vi "Untitled 2.vi"() -> ()   [LabVIEW 2010]
panel:
  in  "VISA resource name":refnum<visa-resource-name>
  out "VISA resource name out":refnum<visa-resource-name>
  out "error out":errorcluster
  in  "error in (no error)":errorcluster
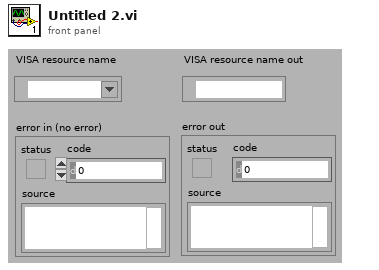
[diagram p1: front panel]
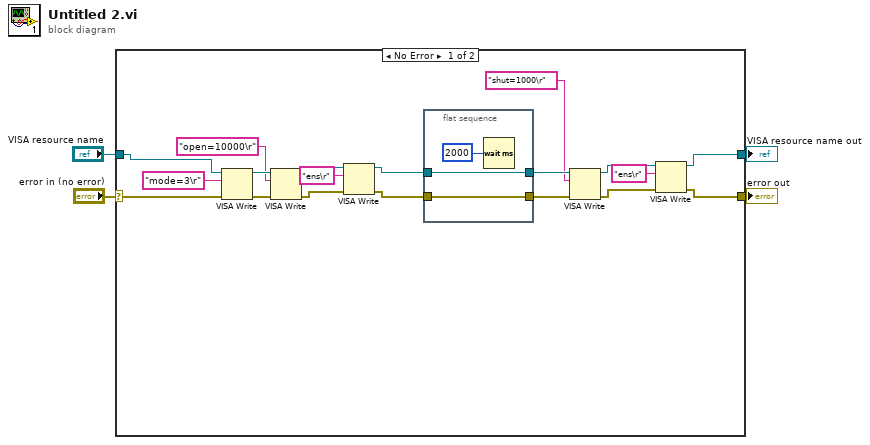
[diagram p0: block diagram]
diagram:
  n1 = case shown="No Error" "error in (no error)" {
    selector: "error in (no error)" -> [w23 w27]
    tunnel: [w6 w27] -> w3
    tunnel: [w8 w28] -> w2
    tunnel: "VISA resource name" -> [w22 w28]
    frame No Error {
      n2 = VISA Write(VISA resource name=w22, write buffer="mode=3\r", error in (no error)=w23) -> (VISA resource name out=w20:refnum<visa-resource-name>, error out=w19:errorcluster)  [unwired: 1 out]
      n3 = VISA Write(VISA resource name=w20, write buffer="open=10000\r", error in (no error)=w19) -> (VISA resource name out=w14:refnum<visa-resource-name>, error out=w13:errorcluster)  [unwired: 1 out]
      n4 = VISA Write(VISA resource name=w14, write buffer="ens\r", error in (no error)=w13) -> (VISA resource name out=w11:refnum<visa-resource-name>, error out=w12:errorcluster)  [unwired: 1 out]
      n5 = flat-sequence {
        tunnel: w11 -> [w25]
        tunnel: [w25] -> w17
        tunnel: w12 -> [w24]
        tunnel: [w24] -> w16
        frame #0 {
          n6 = Wait (ms)(milliseconds to wait=u32 2000) -> ()  [unwired: 1 out]
        }
      }
      n7 = VISA Write(VISA resource name=w17, write buffer="shut=1000\r", error in (no error)=w16) -> (VISA resource name out=w9:refnum<visa-resource-name>, error out=w7:errorcluster)  [unwired: 1 out]
      n8 = VISA Write(VISA resource name=w9, write buffer="ens\r", error in (no error)=w7) -> (VISA resource name out=w8:refnum<visa-resource-name>, error out=w6:errorcluster)  [unwired: 1 out]
    }
    frame Error {
    }
  }
  "error out" <- w3
  "VISA resource name out" <- w2
